vi "SRV_Is Sensor Gauge or Meter.vi"(7 "Sensor View Indicator Names":T1) -> (8 "Gauge or Meter?":bool)   [LabVIEW 2014]
uses:
  SRV_Sensors Names.ctl
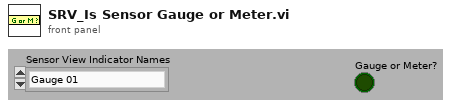
[diagram p1: front panel]
types:
  T1 = typedef "SRV_Sensors Names.ctl" = enum16{"Gauge 01", "Gauge 02", "Gauge 03", "Gauge 04", "Meter 01", "Meter 02", "Meter 03", "Meter 04", "Numeric 01", "Numeric 02", "Numeric 03", "Numeric 04", "Numeric 05", "Numeric 06", "Numeric 07", "Numeric 08", "Boolean 01", "Boolean 02", "Boolean 03", "Boolean 04", "Boolean 05", "Boolean 06", "Boolean 07", "Boolean 08", "Boolean 09", "Boolean 10", "Boolean 11", "Boolean 12", "Boolean 13", "Boolean 14", "Boolean 15", "Boolean 16", "Boolean 17", "Boolean 18", "Boolean 19", "Boolean 20", "Boolean 21", "Boolean 22", "Boolean 23", "Boolean 24", "Boolean 25", "Boolean 26", "Boolean 27", "Boolean 28", "Boolean 29", "Boolean 30", "Boolean 31", "Boolean 32"}
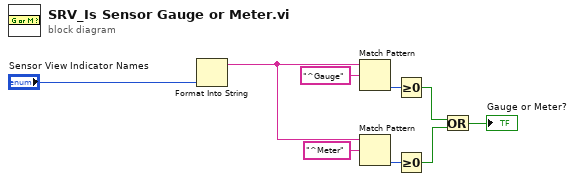
[diagram p0: block diagram]
diagram:
  n1 = Format Into String("Sensor View Indicator Names") -> (resulting string=w1:string)  [unwired: 3 in, 1 out]
  n2 = Match Pattern(string=w1, regular expression="^Gauge") -> (offset past match=w6:i32)  [unwired: 1 in, 3 out]
  n3 = Match Pattern(string=w1, regular expression="^Meter") -> (offset past match=w5:i32)  [unwired: 1 in, 3 out]
  n4 = Greater Or Equal To 0?(x=w6) -> (x >= 0?=w4:bool)
  n5 = Greater Or Equal To 0?(x=w5) -> (x >= 0?=w3:bool)
  n6 = Or(x=w4, y=w3) -> (x .or. y?=→"Gauge or Meter?":bool)
